vi "Overwrite Absolute Delay.vi"(8 "error in (no error)":errorcluster, 10 "Absolute Delay":i32, 11 "User Interface in":refnum<class "User Interface.lvclass">) -> (0 "error out":errorcluster, 3 "User Interface out":refnum<class "User Interface.lvclass">)   [LabVIEW 2016, in "User Interface.lvlib" / "User Interface.lvclass"]
uses:
  User Interface.lvclass
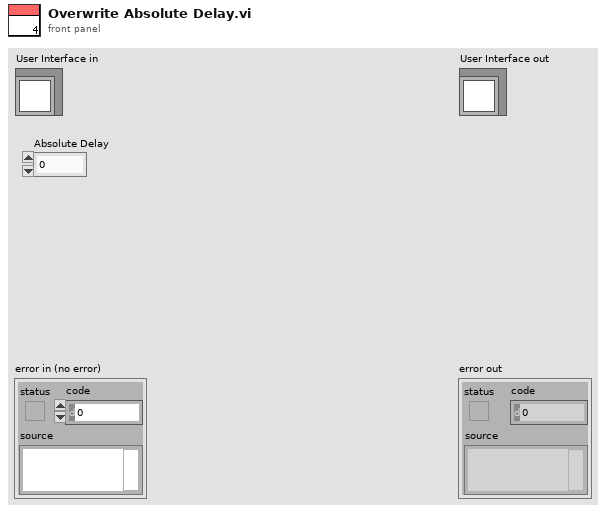
[diagram p1: front panel]
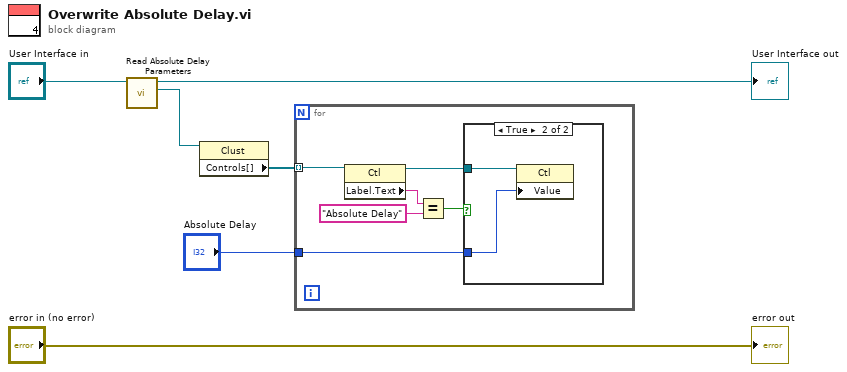
[diagram p0: block diagram]
diagram:
  n1 = call-dynamic "Read Absolute Delay Parameters.vi"("User Interface in"="User Interface in") -> ("Absolute Delay Parameters"=w5:refnum<vi>, "User Interface out"=→"User Interface out":refnum<class "User Interface.lvclass">)  [unwired: 9 in]
  n2 = property class="Clust"(reference=w5) -> ("Controls[]"=w4:refnum<vi>[])  [unwired: 1 in, 2 out]
  n3 = for {
    tunnel: w4 -> [w12] mode=indexing
    tunnel: "Absolute Delay" -> [w7]
    n4 = property class="Ctl"(reference=w12) -> (reference out=w8:refnum<vi>, "Label.Text"=w11:string)  [unwired: 1 in, 1 out]
    n5 = Equal?(x=w11, y="Absolute Delay") -> (x = y?=w9:bool)
    n6 = case shown="True" w9 {
      tunnel: w8 -> [_ w14]
      tunnel: w7 -> [_ w13]
      frame False {
      }
      frame True {
        n7 = property class="Ctl"(reference=w14, "Value"=w13) -> ()  [unwired: 1 in, 2 out]
      }
    }
  }
  "error out" <- "error in (no error)"
